vi "MEMR-Plot Spectra.vi"(0 "Gain spectra in":cluster{"Freq (Hz)":dbl[], "Mag":dbl[][]}[](array[cluster]), 1 "Spectrum":refnum<vi>, 5 "Fmax":dbl=8000.0 format="%#_13g", 7 "Fpeak":dbl, 9 "Noise floor":cluster{"Freq (Hz)":dbl[], dbl[]}[](array[cluster]), 11 "error in (no error)":errorcluster) -> (15 "error out":errorcluster)   [LabVIEW 2015]
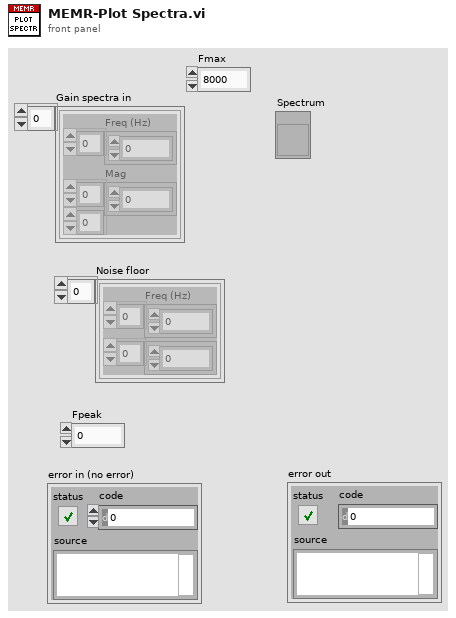
[diagram p1: front panel]
types:
  T1 = enum16{"User", "Prism", "Kelly", "Dark2", "Sequential", "Hue"}
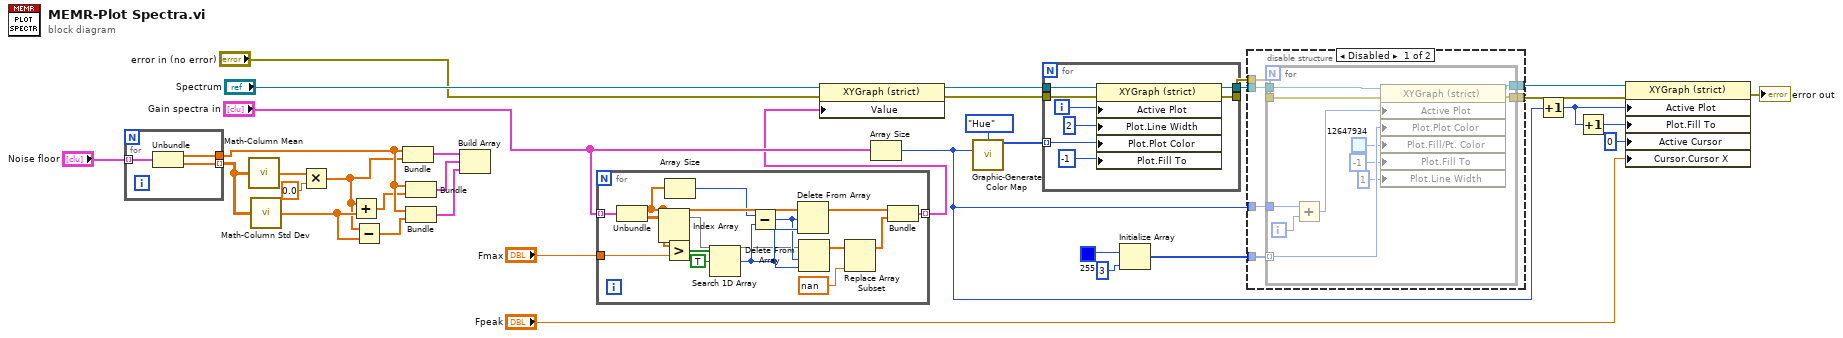
[diagram p0: block diagram]
diagram:
  n1 = for {
    tunnel: "Noise floor" -> [w37] mode=indexing
    tunnel: [w36] -> w19 mode=indexing
    tunnel: [w35] -> w20
    n2 = Unbundle(w37) -> ("Freq (Hz)"=w35:dbl[], w36:dbl[])
  }
  n3 = call "Math-Column Mean.vi"("2D Array"=w19) -> ("Column means"=w11:dbl[])
  n4 = call "Math-Column Std Dev.vi"("2D Array"=w19) -> ("Column means"=w12:dbl[])
  n5 = Multiply(x=w11, y=0.0) -> (x*y=w4:dbl[])
  n6 = Add(x=w4, y=w12) -> (x+y=w13:dbl[])
  n7 = Subtract(x=w4, y=w12) -> (x-y=w14:dbl[])
  n8 = Bundle("Freq (Hz)"=w20, w4) -> (w15:cluster{"Freq (Hz)":dbl[], dbl[]})  [unwired: 1 in]
  n9 = Bundle("Freq (Hz)"=w20, w13) -> (w16:cluster{"Freq (Hz)":dbl[], dbl[]})  [unwired: 1 in]
  n10 = Bundle("Freq (Hz)"=w20, w14) -> (w17:cluster{"Freq (Hz)":dbl[], dbl[]})  [unwired: 1 in]
  n11 = Build Array(w15, w16, w17) -> ()  [unwired: 1 out]
  n12 = for {
    tunnel: "Gain spectra in" -> [w52] mode=indexing
    tunnel: [w47] -> w5 mode=indexing
    tunnel: "Fmax" -> [w38]
    n13 = Unbundle(w52) -> ("Freq (Hz)"=w46:dbl[], "Mag"=w49:dbl[][])
    n14 = Index Array(array=w49) -> (element=w39:dbl[])  [unwired: 2 in]
    n15 = Greater?(x=w46, y=w38) -> (0:w51:bool[])
    n16 = Array Size(array=w46) -> (size(s)=w45:i32)
    n17 = Search 1D Array(1D array=w51, element=TRUE) -> (index of element=w44:i32)  [unwired: 1 in]
    n18 = Subtract(x=w45, y=w44) -> (x-y=w43:i32)
    n19 = Delete From Array(array=w46, length=w43, index=w44) -> (array with subset deleted=w48:dbl[])  [unwired: 1 out]
    n20 = Delete From Array(array=w39, length=w43, index=w44) -> (array with subset deleted=w42:dbl[])  [unwired: 1 out]
    n21 = Replace Array Subset(array=w42, new element=nan) -> (w41:dbl[])  [unwired: 1 in]
    n22 = Bundle("Freq (Hz)"=w48, "Mag"=w41) -> (w47:cluster{"Freq (Hz)":dbl[], "Mag":dbl[]})  [unwired: 1 in]
  }
  n23 = property on="Property Node" class="XYGraph (strict)"(reference="Spectrum", error in="error in (no error)", "Value"=w5) -> (reference out=w10:refnum<vi>, error out=w30:errorcluster)
  n24 = Array Size(array="Gain spectra in") -> (size(s)=w21:i32)
  n25 = call "Graphic-Generate Color Map.vi"("Map"=T1."Hue", "Size"=w21) -> ("Colors"=w31:u32[])  [unwired: 13 in]
  n26 = for {
    tunnel: w31 -> [w58] mode=indexing
    tunnel: w30 -> [w57]
    tunnel: [w56] -> w27
    tunnel: w10 -> [w54]
    tunnel: [w53] -> w9
    i -> [w60]
    n27 = property on="Property Node" class="XYGraph (strict)"(reference=w54, error in=w57, "Active Plot"=w60, "Plot.Line Width"=u8 2, "Plot.Plot Color"=w58, "Plot.Fill To"=i16 -1) -> (reference out=w53:refnum<vi>, error out=w56:errorcluster)
  }
  n28 = Initialize Array(u32 255, 3) -> (w26:u32[])
  n29 = disable-structure shown="Disabled" {
    disable-tunnel: w27 -> [w66 w78]
    disable-tunnel: w26 -> [w65 _]
    disable-tunnel: [w64 w78] -> w25
    disable-tunnel: w21 -> [w63 _]
    disable-tunnel: w9 -> [w62 w79]
    disable-tunnel: [w61 w79] -> w8
    frame Disabled {
      n30 = for {
        tunnel: w66 -> [w77]
        tunnel: w65 -> [w73] mode=indexing
        tunnel: w63 -> [w76]
        tunnel: [w69] -> w64
        tunnel: w62 -> [w68]
        tunnel: [w67] -> w61
        i -> [w75]
        n31 = Add(x=w76, y=w75) -> (x+y=w74:i32)
        n32 = property on="Property Node" class="XYGraph (strict)"(reference=w68, error in=w77, "Active Plot"=w74, "Plot.Plot Color"=w73, "Plot.Fill/Pt. Color"=u32 12647934, "Plot.Fill To"=i16 -1, "Plot.Line Width"=u8 1) -> (reference out=w67:refnum<vi>, error out=w69:errorcluster)
      }
    }
    frame Enabled {
    }
  }
  n33 = Increment(x=w21) -> (x+1=w24:i32)
  n34 = Increment(x=w24) -> (x+1=w23:i32)
  n35 = property on="Property Node" class="XYGraph (strict)"(reference=w8, error in=w25, "Active Plot"=w24, "Plot.Fill To"=w23, "Active Cursor"=u32 0, "Cursor.Cursor X"="Fpeak") -> (error out=→"error out":errorcluster)  [unwired: 1 out]
